vi "cnc-rpm.vi"(1 "speed in":i32(listbox)) -> (0 "rpm out":dbl(knob) scale=0.0..10.0)   [LabVIEW 2026]
uses:
  <vilib>/numeric/Random Number (Range) DBL.vi
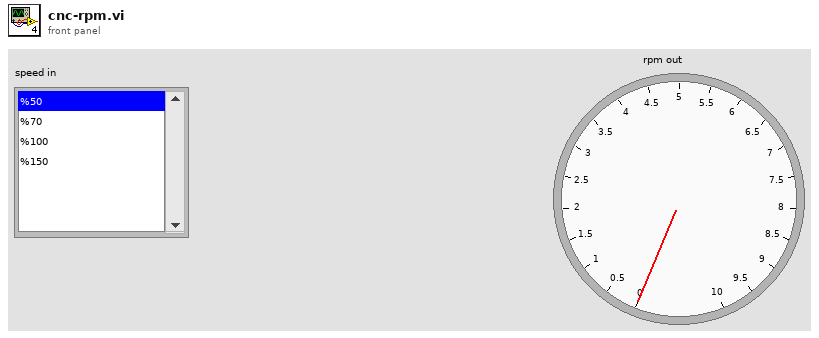
[diagram p1: front panel]
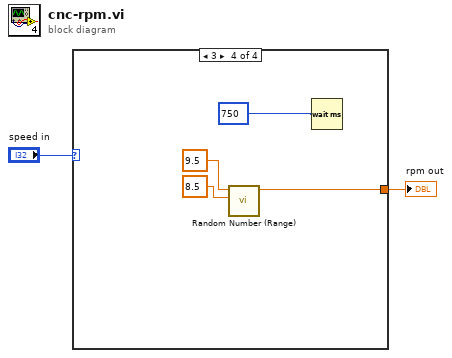
[diagram p0: block diagram]
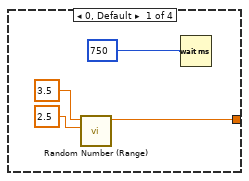
[diagram p2: hidden frame]
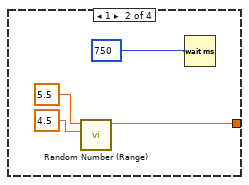
[diagram p3: hidden frame]
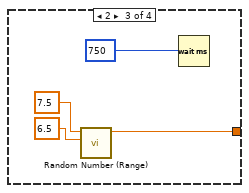
[diagram p4: hidden frame]
diagram:
  n1 = case shown="3" "speed in" {
    tunnel: [w4 w8 w12 w16] -> w1
    frame 0, Default {
      n2 = call-poly <vilib>:"Random Number (Range).vi"("lower bound (0)"=2.5, "upper bound (100)"=3.5 ("lower bound (0)")) -> ("number"=w4:dbl)  [unwired: 9 in]
      n3 = Wait (ms)(milliseconds to wait=u32 750) -> ()  [unwired: 1 out]
    }
    frame 1 {
      n4 = call-poly <vilib>:"Random Number (Range).vi"("lower bound (0)"=4.5, "upper bound (100)"=5.5 ("lower bound (0)")) -> ("number"=w8:dbl)  [unwired: 9 in]
      n5 = Wait (ms)(milliseconds to wait=u32 750) -> ()  [unwired: 1 out]
    }
    frame 2 {
      n6 = call-poly <vilib>:"Random Number (Range).vi"("lower bound (0)"=6.5, "upper bound (100)"=7.5 ("lower bound (0)")) -> ("number"=w12:dbl)  [unwired: 9 in]
      n7 = Wait (ms)(milliseconds to wait=u32 750) -> ()  [unwired: 1 out]
    }
    frame 3 {
      n8 = call-poly <vilib>:"Random Number (Range).vi"("lower bound (0)"=8.5, "upper bound (100)"=9.5 ("lower bound (0)")) -> ("number"=w16:dbl)  [unwired: 9 in]
      n9 = Wait (ms)(milliseconds to wait=u32 750) -> ()  [unwired: 1 out]
    }
  }
  "rpm out" <- w1
